vi "GetIniScripts.vi"(8 "ErrorArray":errorcluster[](array[cluster]), 10 "ModIndexArray":T1[](array[typedef])=[2, 0, 1] items=["Sync"=2, "Wfrm"=0, "FGen"=1], 11 "TestBase.lvclass":refnum<class "TestBase.lvclass">) -> (0 "ErrorArray":errorcluster[](array[cluster]), 2 "Script":string[](array[string]), 3 "TestBase.lvclass":refnum<class "TestBase.lvclass">)   [LabVIEW 2014, in "TestBase.lvclass"]
uses:
  TestBase.lvclass
  TypeDefs/rngModIndex.ctl
  TestBase.lvclass/TestBase.ctl
  Accessors/Read ErrorSeverity.vi
  Accessors/Read PluginPathArray.vi
  Accessors/Read PluginIndex.vi
  <vilib>/Utility/error.llb/Error Cluster From Error Code.vi
  <vilib>/ErrorRing/Error Ring.xnode
  <vilib>/Utility/config.llb/NI_LVConfig.lvlib
  <userlib>/NIST/NISTErrorLib/NISTErrorLib.lvlib
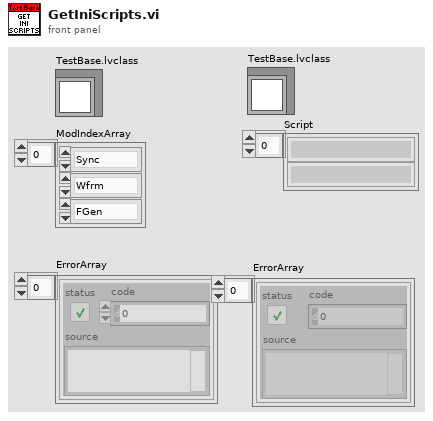
[diagram p1: front panel]
types:
  T1 = typedef "TestBase.lvclass/rngModIndex.ctl" = u16
  T2 = typedef "NI_LVConfig.lvlib/Config Data RefNum.ctl" = refnum<k1>
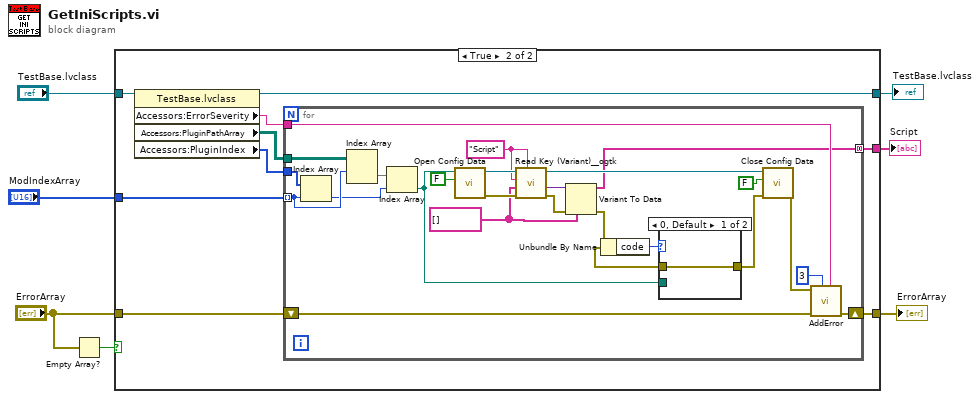
[diagram p0: block diagram]
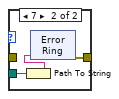
[diagram p3: hidden frame]
diagram:
  n1 = Empty Array?(array="ErrorArray") -> (empty?=w7:bool)
  n2 = case shown="True" w7 {
    tunnel: "ErrorArray" -> [w9 w15]
    tunnel: [w9 w13] -> w5
    tunnel: "TestBase.lvclass" -> [w8 w18]
    tunnel: [w8 w11] -> w3
    tunnel: [_ w12] -> w2
    tunnel: "ModIndexArray" -> [_ w10]
    frame False {
    }
    frame True {
      n3 = property class="TestBase.lvclass"(reference=w18) -> (reference out=w11:refnum<class "TestBase.lvclass">, "Accessors:ErrorSeverity"=w14:string, "Accessors:PluginPathArray"=w17:path[][], "Accessors:PluginIndex"=w16:u32[])  [unwired: 1 in, 1 out]
      n4 = for {
        tunnel: w17 -> [w23]
        tunnel: w16 -> [w22]
        shift-right: [w27] -> w13
        shift-left: w15 -> [w31]
        tunnel: w14 -> [w30]
        tunnel: [w26] -> w12 mode=concatenating
        tunnel: w10 -> [w20] mode=indexing
        w24 = "Script" ("section")
        w37 = string[] []
        n5 = Index Array(array=w22, index=w20) -> (element=w19:u32)
        n6 = Index Array(array=w23, index (row)=w20) -> (element=w21:path[])  [unwired: 1 in]
        n7 = Index Array(array=w21, index=w19) -> (element=w25:path)
        n8 = call <vilib>:"Open Config Data.vi"("create file if necessary (T)"=FALSE, "configuration file path"=w25) -> ("error out"=w41:errorcluster, "refnum"=w40:T2)  [unwired: 7 in, 1 out]
        n9 = call <userlib>:"Read Key (Variant)__ogtk.vi"("section"=w24, "error in (no error)"=w41, "type"=w37, "key (optional)"=w24, "refnum"=w40) -> ("error out"=w38:errorcluster, "key-value"=w39:variant, "refnum out"=w34:T2)  [unwired: 3 in, 1 out]
        n10 = Variant To Data(error in=w38, type=w37, Variant=w39) -> (data=w26:string[], error out=w35:errorcluster)
        n11 = Unbundle By Name(w35) -> ("code"=w36:i32)
        n12 = case shown="0, Default" w36 {
          tunnel: w35 -> [w43 _]
          tunnel: [w43 w46] -> w32
          tunnel: w25 -> [_ w45]
          frame 0, Default {
          }
          frame 7 {
            n13 = Path To String(path=w45) -> (string=w44:string)
            n14 = xnode "Error Ring"("parameter 0"=w44) -> ("error out"=w46:errorcluster)
          }
        }
        n15 = call <vilib>:"Close Config Data.vi"("error in (no error)"=w32, "write file if changed (T)"=FALSE, "refnum"=w34) -> ("error out"=w28:errorcluster)  [unwired: 7 in, 1 out]
        n16 = call <userlib>:"AddError.vi"("Severity"=w30, "Priority"=u8 3, "ErrorArray"=w31, "error in (no error)"=w28) -> ("ErrorArray"=w27:errorcluster[])  [unwired: 6 in, 1 out]
      }
    }
  }
  "ErrorArray" <- w5
  "TestBase.lvclass" <- w3
  "Script" <- w2
